vi "IsSatisfied.vi"(10 "Product":refnum<class "Product.lvclass">, 11 "BlahSpec":refnum<class "BlahSpec.lvclass">) -> (2 "IsSatisfied":bool)   [LabVIEW 2020, in "BlahSpec.lvclass"]
uses:
  BlahSpec.lvclass
  Product/Product.lvclass
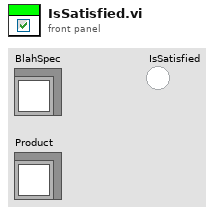
[diagram p1: front panel]
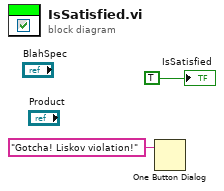
[diagram p0: block diagram]
diagram:
  n1 = One Button Dialog(message="Gotcha! Liskov violation!") -> ()  [unwired: 1 in, 1 out]
  "IsSatisfied" <- TRUE ("IsSatisfied")
